vi "startstop.vi"(1 "Input":variant, 2 "Message":u16(ring) items=["GetText", "Click"], 3 "Handle":u64) -> (0 "Output":variant)   [LabVIEW 2014]
uses:
  user32.dll
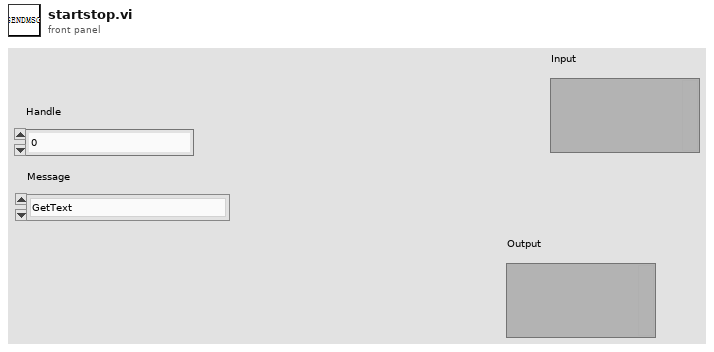
[diagram p1: front panel]
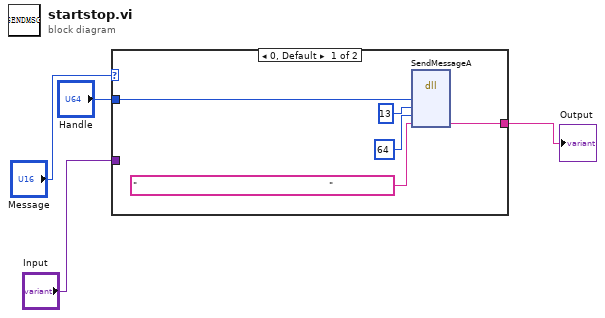
[diagram p0: block diagram]
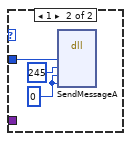
[diagram p2: hidden frame]
diagram:
  n1 = case shown="0, Default" "Message" {
    tunnel: "Handle" -> [w9 w12]
    tunnel: [w5 _] -> w3
    tunnel: "Input" -> [_ _]
    frame 0, Default {
      n2 = dll-call lib="user32.dll" fn="SendMessageA"("arg3"=w9, "arg4"=13, "arg1"=u64 64, "arg2"="                                                                ") -> ("arg2"=w5:string)  [unwired: 7 in, 2 out]
    }
    frame 1 {
      w10 = i16 0 ("arg1")
      n3 = dll-call lib="user32.dll" fn="SendMessageA"("arg3"=w12, "arg4"=245, "arg1"=w10, "arg2"=w10) -> ()  [unwired: 8 in, 2 out]
    }
  }
  "Output" <- w3
